vi "Generate Command Frame Vectors.vi"(0 "RFFE Reg0Write Command in":refnum<class "RFFE Reg0Write Command.lvclass">, 11 "error in (no error)":errorcluster) -> (4 "RFFE Reg0Write Command out":refnum<class "RFFE Reg0Write Command.lvclass">, 6 "Vector Statements":string[](array[string]), 15 "error out":errorcluster)   [LabVIEW 2018, in "MIPI RFFE API.lvlib" / "RFFE Reg0Write Command.lvclass"]
uses:
  RFFE Reg0Write Command.lvclass
  Command/RFFE Command.lvclass
  MIPI RFFE API.lvlib
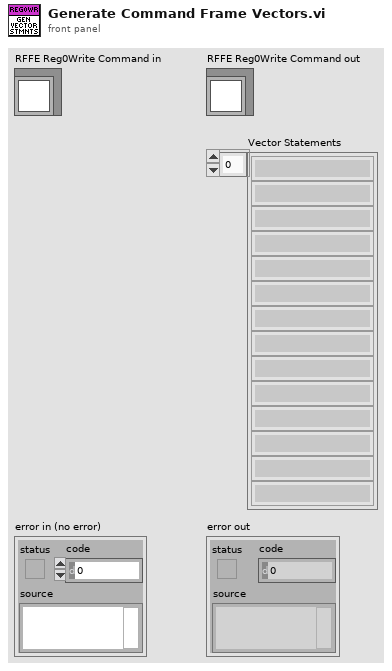
[diagram p1: front panel]
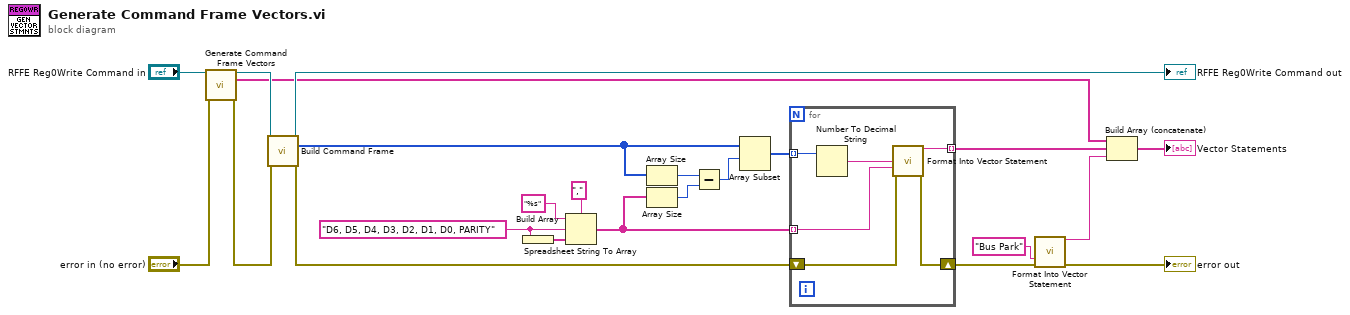
[diagram p0: block diagram]
diagram:
  w19 = "D6, D5, D4, D3, D2, D1, D0, PARITY"
  n1 = call-parent "Generate Command Frame Vectors.vi"("RFFE Command in"="RFFE Reg0Write Command in", "error in (no error)"="error in (no error)") -> ("RFFE Command out"=w14:refnum<class "RFFE Reg0Write Command.lvclass">, "Command Frame Vectors"=w6:string[], "error out"=w13:errorcluster)  [unwired: 11 in]
  n2 = call-dynamic "Build Command Frame.vi"("RFFE Reg0Write Command in"=w14, "error in (no error)"=w13) -> ("RFFE Reg0Write Command out"=→"RFFE Reg0Write Command out":refnum<class "RFFE Reg0Write Command.lvclass">, "Command Frame"=w10:u8[], "error out"=w15:errorcluster)  [unwired: 11 in]
  n3 = Build Array(w19) -> (w18:string[])
  n4 = Spreadsheet String To Array(delimiter (Tab)=",", format string="%s", spreadsheet string=w19, array type (2D Dbl)=w18) -> (array=w12:string[])
  n5 = Array Size(array=w10) -> (size(s)=w9:i32)
  n6 = Array Size(array=w12) -> (size(s)=w8:i32)
  n7 = Subtract(x=w9, y=w8) -> (x-y=w7:i32)
  n8 = Array Subset(array=w10, index=w7) -> (w11:u8[])  [unwired: 1 in]
  n9 = for {
    tunnel: w11 -> [w29] mode=indexing
    shift-right: [w25] -> w4
    shift-left: w15 -> [w26]
    tunnel: w12 -> [w27] mode=indexing
    tunnel: [w24] -> w5 mode=indexing
    n10 = Number To Decimal String(number=w29) -> (decimal integer string=w28:string)  [unwired: 1 in]
    n11 = call "Format Into Vector Statement.vi"("DATA (0)"=w28, "Comment"=w27, "error in (no error)"=w26) -> ("Vector Statement"=w24:string, "error out"=w25:errorcluster)  [unwired: 11 in]
  }
  n12 = call "Format Into Vector Statement.vi"("Comment"="Bus Park", "error in (no error)"=w4) -> ("Vector Statement"=w1:string, "error out"=→"error out":errorcluster)  [unwired: 12 in]
  n13 = Build Array (concatenate)(w6, w5, w1) -> (→"Vector Statements":string[])
